vi "Query.vi"(8 "error in":errorcluster, 10 "Write in":string, 11 "57XX in":refnum<class "57XX.lvclass">) -> (0 "error out":errorcluster, 2 "Read out":string, 3 "57XX out":refnum<class "57XX.lvclass">)   [LabVIEW 2019, in "57XX.lvlib" / "57XX.lvclass"]
uses:
  Library/57XX.lvclass
  Library/57XX.lvclass/57XX.ctl
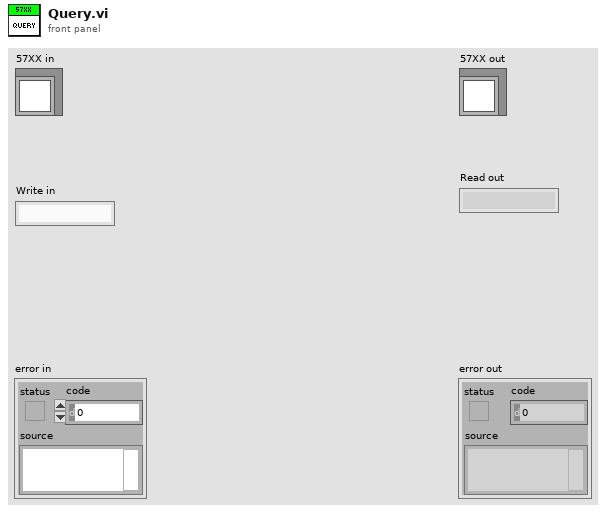
[diagram p1: front panel]
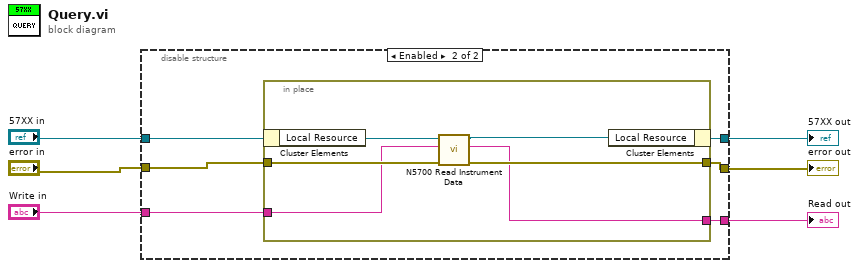
[diagram p0: block diagram]
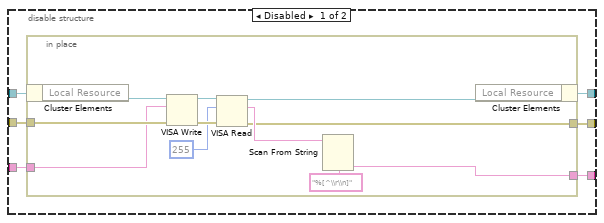
[diagram p2: hidden frame]
diagram:
  n1 = disable-structure shown="Enabled" {
    disable-tunnel: [w7 w29] -> w6
    disable-tunnel: "Write in" -> [w12 w28]
    disable-tunnel: "57XX in" -> [w11 w27]
    disable-tunnel: [w10 w26] -> w3
    disable-tunnel: "error in" -> [w9 w25]
    disable-tunnel: [w8 w24] -> w1
    frame Disabled {
      n2 = in-place {
        in-place-border: w9 -> [w17]
        in-place-border: w12 -> [w16]
        in-place-border: [w14] -> w8
        in-place-border: [w13] -> w7
        n3 = in-place-cluster #1(w11) -> ("Local Resource"=w18:refnum<visa-resource-name>)
        n4 = VISA Write(VISA resource name=w18, write buffer=w16, error in (no error)=w17) -> (VISA resource name out=w23:refnum<visa-resource-name>, error out=w22:errorcluster)  [unwired: 1 out]
        n5 = VISA Read(VISA resource name=w23, byte count=u32 255 ("byte count (0)"), error in (no error)=w22) -> (VISA resource name out=w15:refnum<visa-resource-name>, read buffer=w21:string, error out=w14:errorcluster)  [unwired: 1 out]
        n6 = Scan From String(format string="%[^\\r\\n]", input string=w21) -> (output 1=w13:string)  [unwired: 3 in, 3 out]
        n7 = in-place-cluster #1("Local Resource"=w15) -> (w10:refnum<class "57XX.lvclass">)
      }
    }
    frame Enabled {
      n8 = in-place {
        in-place-border: w25 -> [w33]
        in-place-border: w28 -> [w31]
        in-place-border: [w32] -> w24
        in-place-border: [w30] -> w29
        n9 = in-place-cluster #2(w27) -> ("Local Resource"=w35:refnum<visa-resource-name>)
        n10 = call <instrlib>:"N5700 Read Instrument Data.vi"("error"=w33, "Query"=w31, "VISA"=w35) -> ("error out"=w32:errorcluster, "Response"=w30:string, "VISA out"=w34:refnum<visa-resource-name>)  [unwired: 2 in, 1 out]
        n11 = in-place-cluster #2("Local Resource"=w34) -> (w26:refnum<class "57XX.lvclass">)
      }
    }
  }
  "error out" <- w1
  "57XX out" <- w3
  "Read out" <- w6
